vi "DWDT Analog to Digital.vi"(6 "data format (offset binary)":u16(ring)=1 items=["unsigned binary", "offset binary", "2's complement"], 7 "compress digital (T)":bool=TRUE, 8 "error in (no error)":errorcluster, 9 "full-scale range (pk-pk)":dbl=2.0, 10 "resolution (16 bit)":i32=16, 11 "analog waveform":waveform(dbl)) -> (0 "error out":errorcluster, 1 "full-scale range (out)":dbl, 2 "resolution (out)":i32=16, 3 "digital waveform":digitalwaveform(waveform)={"t0"=timestamp(0 s since 1904-01-01), "dt"=0.0, "Y"={"transitions"=[], "data"=[]}, "error"={"status"=FALSE, "code"=37421928, "source"=""}})   [LabVIEW 2020]
doc: "Converts <B>analog waveform</B> to a digital waveform or digital data. You must manually select the polymorphic instance you want to use."
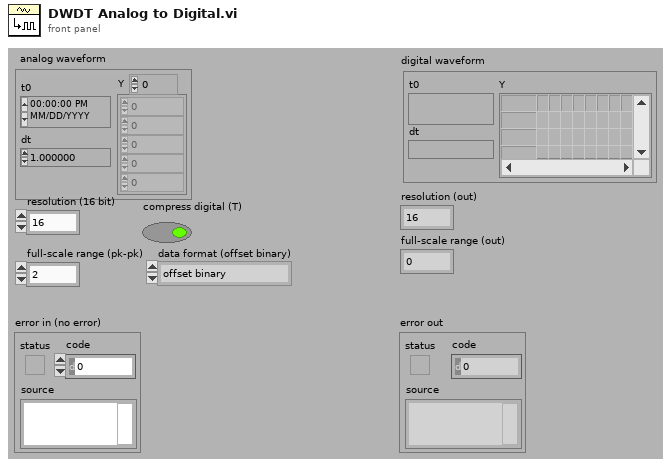
[diagram p1: front panel]
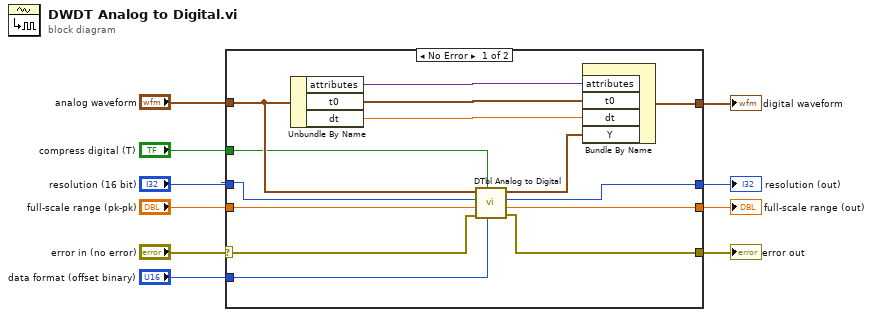
[diagram p0: block diagram]
diagram:
  n1 = case shown="No Error" "error in (no error)" {
    selector: "error in (no error)" -> [w19 w27]
    tunnel: "analog waveform" -> [w20 _]
    tunnel: [w24 _] -> w8
    tunnel: [w13 w27] -> w7
    tunnel: "resolution (16 bit)" -> [w18 w26]
    tunnel: "compress digital (T)" -> [w17 _]
    tunnel: "data format (offset binary)" -> [w16 _]
    tunnel: [w14 w26] -> w4
    tunnel: "full-scale range (pk-pk)" -> [w12 w25]
    tunnel: [w11 w25] -> w2
    frame No Error {
      n2 = Unbundle By Name(w20) -> ("attributes"=w22:variant, "t0"=w21:timestamp, "dt"=w23:dbl)
      n3 = call "DTbl Analog to Digital.vi"("data format (offset binary)"=w16, "compress digital (T)"=w17, "error in (no error)"=w19, "full-scale range (pk-pk)"=w12, "resolution (16 bit)"=w18, "analog waveform"=w20) -> ("error out"=w13:errorcluster, "full-scale range (out)"=w11:dbl, "resolution (out)"=w14:i32, "digital data"=w15:digitaldata)  [unwired: 2 in]
      n4 = Bundle By Name("attributes"=w22, "t0"=w21, "dt"=w23, "Y"=w15) -> (w24:digitalwaveform)  [unwired: 1 in]
    }
    frame Error {
      # "Return empty array\non input error."
    }
  }
  "error out" <- w7
  "digital waveform" <- w8
  "resolution (out)" <- w4
  "full-scale range (out)" <- w2
